vi "Get Histogram Fit Axis v2.vi"(8 "Bin Location (Left)":T1, 10 "Histogram Values":dbl[](array[numeric]), 11 "Histogram Axis":dbl[](array[numeric])) -> (0 "Step Size":dbl, 1 "Uniformly spaced data?":bool, 2 "Ordered Axis Histogram Values":dbl[](array[numeric]), 3 "Ordered Histogram Axis":dbl[](array[numeric]), 4 "Step Sizes":dbl[](array[numeric]), 5 "Truncated?":bool)   [LabVIEW 2019]
uses:
  Histogram Bin Position.ctl
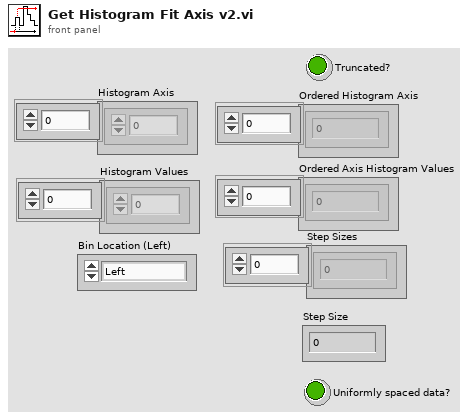
[diagram p1: front panel]
types:
  T1 = typedef "Histogram Bin Position.ctl" = enum16{"Left", "Center", "Right"}
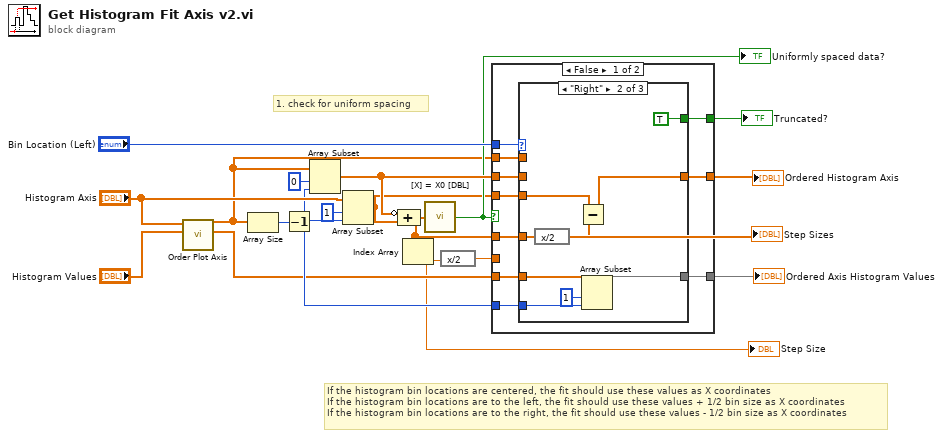
[diagram p0: block diagram]
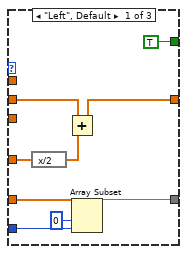
[diagram p2: hidden frame]
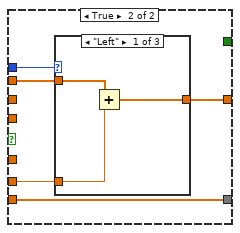
[diagram p4: hidden frame]
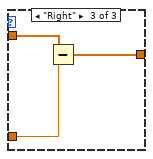
[diagram p6: hidden frame]
diagram:
  # "1. check for uniform spacing"
  # "If the histogram bin locations are centered, the fit should use these values as X coordinates\nIf the histogram bin locations are to the left, the fit should use these values + 1/2 bin size as X coordinates\nIf the histogram bin locations are to the right, the fit should use these values - 1/2 bin size as X coordinates"
  n1 = call "Order Plot Axis.vi"("Plot Values"="Histogram Values", "Plot Axis"="Histogram Axis") -> ("Ordered Axis Plot Values"=w3:dbl[], "Ordered Plot Axis"=w2:dbl[])  [unwired: 8 in]
  n2 = Array Size(array=w2) -> (size(s)=w15:i32)
  n3 = Decrement(x=w15) -> (x-1=w6:i32)
  n4 = Array Subset(array=w2, index=0, length=w6) -> (w13:dbl[])
  n5 = Array Subset(array="Histogram Axis", index=1, length=w6) -> (w5:dbl[])
  n6 = Compound Arithmetic op=ADD(invert w13, w5) -> (w10:dbl[])
  "Step Sizes" <- w10
  n7 = Index Array(array=w10) -> (element=w1:dbl)  [unwired: 1 in]
  "Step Size" <- w1
  n8 = call "[X] = X0 [DBL].vi"("X"=w10) -> ("All Identical?"=w8:bool)  [unwired: 14 in]
  "Uniformly spaced data?" <- w8
  n9 = expression code="x/2"(w1) -> (w4:dbl)
  n10 = case shown="False" w8 {
    tunnel: "Bin Location (Left)" -> [w28 w53]
    tunnel: [w27 w52] -> w17
    tunnel: w13 -> [w21 _]
    tunnel: w3 -> [w25 w51]
    tunnel: [w24 w51] -> w11
    tunnel: w10 -> [w22 _]
    tunnel: w2 -> [w26 w50]
    tunnel: w4 -> [_ w49]
    tunnel: [w23 _] -> w7
    tunnel: w6 -> [w20 _]
    tunnel: w5 -> [w19 _]
    frame False {
      n11 = case shown="\"Right\"" w28 {
        tunnel: [w33 w43 w48] -> w27
        tunnel: w26 -> [_ _ w48]
        tunnel: w25 -> [w32 w42 w47]
        tunnel: [w29 w39 w47] -> w24
        tunnel: [TRUE ("Truncated?") TRUE ("Truncated?") _] -> w23
        tunnel: w22 -> [w36 w45 _]
        tunnel: w21 -> [w35 _ _]
        tunnel: w20 -> [w30 w40 _]
        tunnel: w19 -> [_ w38 _]
        frame "Left", Default {
          n12 = expression code="x/2"(w36) -> (w34:dbl[])
          n13 = Add(x=w35, y=w34) -> (x+y=w33:dbl[])
          n14 = Array Subset(array=w32, index=0, length=w30) -> (w29:dbl[])
        }
        frame "Right" {
          n15 = expression code="x/2"(w45) -> (w44:dbl[])
          n16 = Subtract(x=w38, y=w44) -> (x-y=w43:dbl[])
          n17 = Array Subset(array=w42, index=1, length=w40) -> (w39:dbl[])
        }
        frame "Center" {
        }
      }
    }
    frame True {
      n18 = case shown="\"Left\"" w53 {
        tunnel: w49 -> [w56 _ w59]
        tunnel: [w55 w57 w60] -> w52
        tunnel: w50 -> [w54 w57 w58]
        frame "Left" {
          n19 = Add(x=w54, y=w56) -> (x+y=w55:dbl[])
        }
        frame "Center", Default {
        }
        frame "Right" {
          n20 = Subtract(x=w58, y=w59) -> (x-y=w60:dbl[])
        }
      }
    }
  }
  "Ordered Histogram Axis" <- w17
  "Ordered Axis Histogram Values" <- w11
  "Truncated?" <- w7
